vi "Get Location.vi"(8 "error in (no error)":errorcluster, 11 "MouseEventArgs in":refnum<class "MouseEventArgs.lvclass">) -> (0 "error out":errorcluster, 2 "Location":cluster{"X":i32, "Y":i32}, 3 "MouseEventArgs out":refnum<class "MouseEventArgs.lvclass">)   [LabVIEW 2023, in "SourceGrid.lvlib" / "MouseEventArgs.lvclass"]
doc: "Gets the location of the mouse during the generating mouse event."
uses:
  MouseEventArgs.lvclass
  MouseEventArgs.lvclass/MouseEventArgs.ctl
  System.Windows.Forms
  System.Drawing
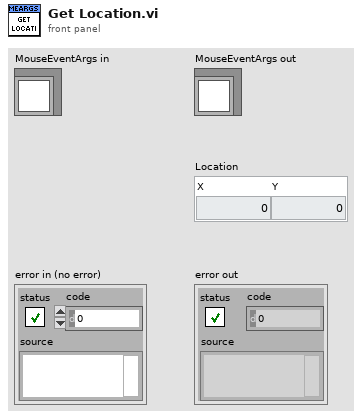
[diagram p1: front panel]
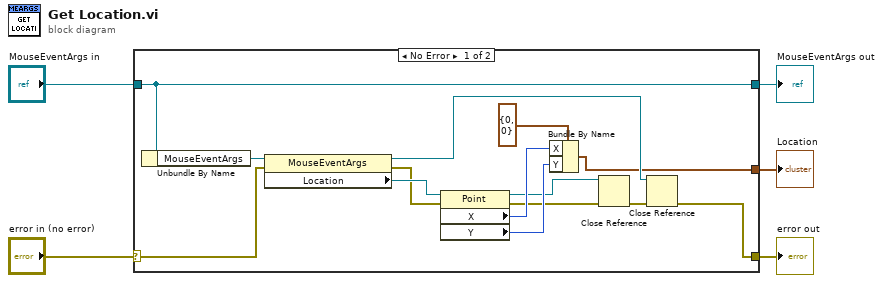
[diagram p0: block diagram]
diagram:
  n1 = case shown="No Error" "error in (no error)" {
    selector: "error in (no error)" -> [w10 w20]
    tunnel: [w7 w20] -> w4
    tunnel: [w19 w21] -> w2
    tunnel: "MouseEventArgs in" -> [w19 w21]
    tunnel: [w6 _] -> w1
    frame No Error {
      n2 = Unbundle By Name(w19) -> ("MouseEventArgs"=w11:refnum<k24>)
      n3 = property class="MouseEventArgs"(reference=w11, error in=w10) -> (reference out=w8:refnum<k24>, error out=w14:errorcluster, "Location"=w18:refnum<k24>)
      n4 = property class="Point"(reference=w18, error in=w14) -> (reference out=w12:refnum<k24>, error out=w13:errorcluster, "X"=w16:i32, "Y"=w15:i32)
      n5 = Bundle By Name(cluster=cluster{"X":i32, "Y":i32} {"X"=0, "Y"=0} ("Location"), "X"=w16, "Y"=w15) -> (w6:cluster{"X":i32, "Y":i32})
      n6 = Close Reference(reference=w12, error in (no error)=w13) -> (error out=w9:errorcluster)
      n7 = Close Reference(reference=w8, error in (no error)=w9) -> (error out=w7:errorcluster)
    }
    frame Error {
    }
  }
  "error out" <- w4
  "MouseEventArgs out" <- w2
  "Location" <- w1
